vi "Init.vi"(0 "EK-P4.lvclass":refnum<class "EK-P4.lvclass">, 5 "VISA Refnum in":refnum<visa-resource-name>, 7 "Measurement interval [ms] in":u16=1 caption="Measurement interval [ms]", 9 "address (USB SensorCable)":u8, 11 "error in (no error)":errorcluster) -> (4 "EK-P4.lvclass 2":refnum<class "EK-P4.lvclass">, 6 "FoundI2cAddresses":u8[](array[numeric]) caption="Rx data" format="%02x", 15 "error out":errorcluster)   [LabVIEW 2016, in "EK-P4.lvclass"]
doc: "initializes connection to the Ek-P4 sensirion board using I2C"
uses:
  EK-P4.lvclass
  UsbScShdlc_Sensirion/control/modeReadWrite_UsbScShdlc_Sensirion.ctl
  UsbScShdlc_Sensirion/control/SensorVoltage_UsbScShdlc_Sensirion.ctl
  UsbScShdlc_Sensirion/control/SensorType_UsbScShdlc_Sensirion.ctl
  EK-P4.lvclass/EK-P4.ctl
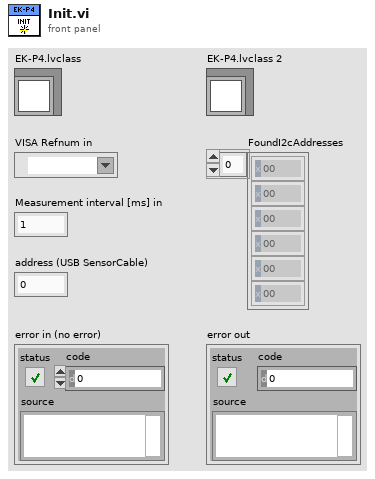
[diagram p1: front panel]
types:
  T1 = typedef "SensorType_UsbScShdlc_Sensirion.ctl" = enum16{"SF04 Flow Sensor", "Humidity Sensor", "SF05 Flow Sensor", "SF06 Flow Sensor"}
  T2 = typedef "SensorVoltage_UsbScShdlc_Sensirion.ctl" = enum16{"3.3V", "5.0V"}
  T3 = typedef "modeReadWrite_UsbScShdlc_Sensirion.ctl" = bool
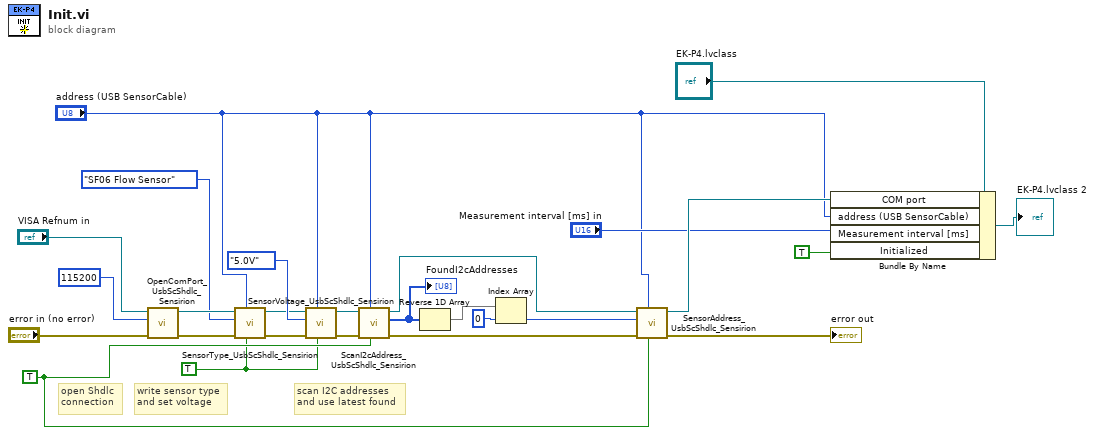
[diagram p0: block diagram]
diagram:
  w17 = TRUE ("range")
  w14 = T3 TRUE ("mode")
  # "scan I2C addresses \nand use latest found"
  # "write sensor type\nand set voltage"
  # "open Shdlc\nconnection"
  n1 = call "OpenComPort_UsbScShdlc_Sensirion.vi"("error in (no error)"="error in (no error)", "baud rate (115200)"=u32 115200, "COM port"="VISA Refnum in") -> ("error out"=w13:errorcluster, "COM port out"=w12:refnum<visa-resource-name>)  [unwired: 7 in]
  n2 = call "SensorType_UsbScShdlc_Sensirion.vi"("mode"=w14, "address"="address (USB SensorCable)", "error in (no error)"=w13, "SensorType"=SensorType_UsbScShdlc_Sensirion."SF06 Flow Sensor", "COM port"=w12) -> ("error out"=w9:errorcluster, "COM port out"=w10:refnum<visa-resource-name>)  [unwired: 4 in, 1 out]
  n3 = call "SensorVoltage_UsbScShdlc_Sensirion.vi"("mode"=w14, "address"="address (USB SensorCable)", "error in (no error)"=w9, "SensorVoltage"=SensorVoltage_UsbScShdlc_Sensirion."5.0V", "COM port"=w10) -> ("error out"=w22:errorcluster, "COM port out"=w23:refnum<visa-resource-name>)  [unwired: 4 in, 1 out]
  n4 = call "ScanI2cAddress_UsbScShdlc_Sensirion.vi"("range"=w17, "address"="address (USB SensorCable)", "error in (no error)"=w22, "COM port"=w23) -> ("error out"=w15:errorcluster, "FoundI2cAddresses"=w18:u8[], "COM port out"=w16:refnum<visa-resource-name>)  [unwired: 5 in]
  "FoundI2cAddresses" <- w18
  n5 = Reverse 1D Array(array=w18) -> (reversed array=w19:u8[])
  n6 = Index Array(array=w19, index=0) -> (element=w21:u8)
  n7 = call "SensorAddress_UsbScShdlc_Sensirion.vi"("mode"=w17, "address"="address (USB SensorCable)", "error in (no error)"=w15, "SensorAddress"=w21, "COM port"=w16) -> ("error out"=→"error out":errorcluster, "COM port out"=w24:refnum<visa-resource-name>)  [unwired: 4 in, 1 out]
  n8 = Bundle By Name(cluster="EK-P4.lvclass", "COM port"=w24, "address (USB SensorCable)"="address (USB SensorCable)", "Measurement interval [ms]"="Measurement interval [ms] in", "Initialized"=TRUE) -> (→"EK-P4.lvclass 2":refnum<class "EK-P4.lvclass">)
